vi "Read_CSV_Files_9205x3.vi"() -> ()   [LabVIEW 2018]
uses:
  <vilib>/express/express analysis/Spectral/Block/exnSpectralBlock spectral measurements RMS poly.vi
  <vilib>/express/express analysis/Spectral/Block/exnSpectralBlock spectral measurements RMS DDT.vi
  <vilib>/ErrorRing/Error Ring.xnode
  <vilib>/express/express analysis/Spectral/XNode/ExpressSpectralMeasurementsBlockNode.xnode
panel:
  in  "FFT Mode":bool
  in  "Rechose":bool
  in  "Rescan":bool
  in  "Data Connect":bool
  in  "FFT export":bool
  in  "Filenames":i32(listbox)
  out "error out":errorcluster
  out "Timedomain":dynamicdata(graph)
  out "FFT":dynamicdata(graph)
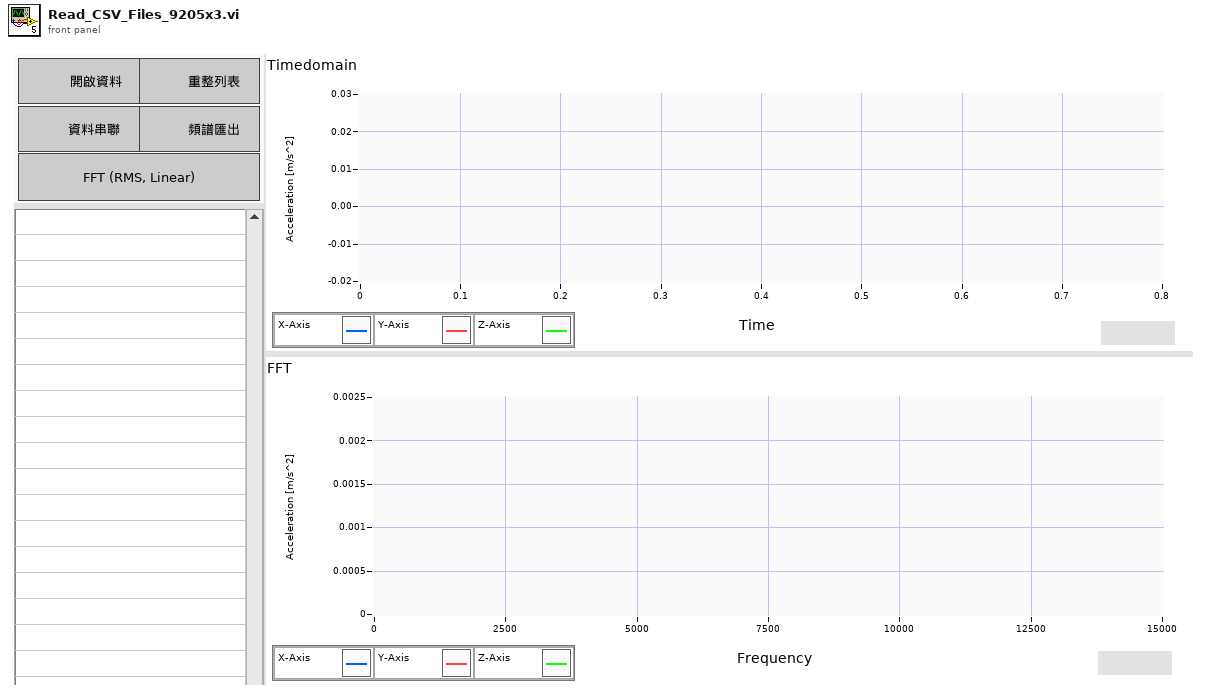
[diagram p1: front panel]
types:
  T1 = cluster{"averaging mode":u16, "weighting mode":u16, "number of averages":u32}
  T2 = cluster{"dB On (F)":bool, "unwrap phase (F)":bool, "convert to degree (F)":bool}
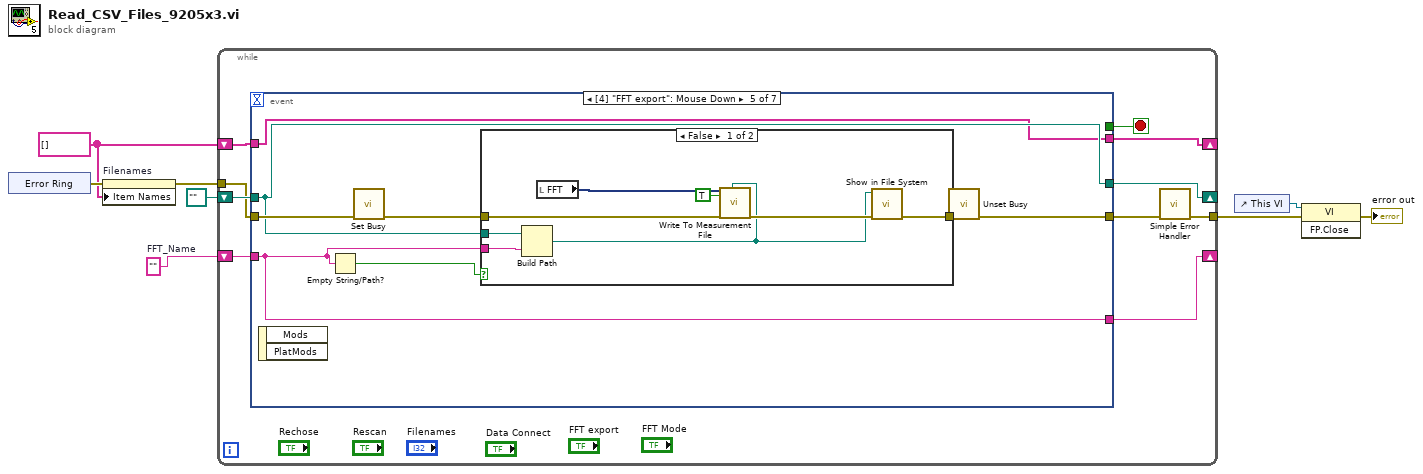
[diagram p0: block diagram]
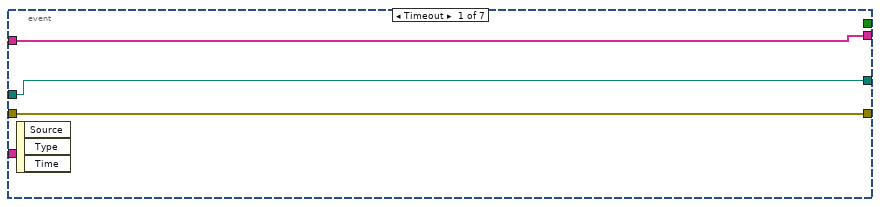
[diagram p2: hidden frame]
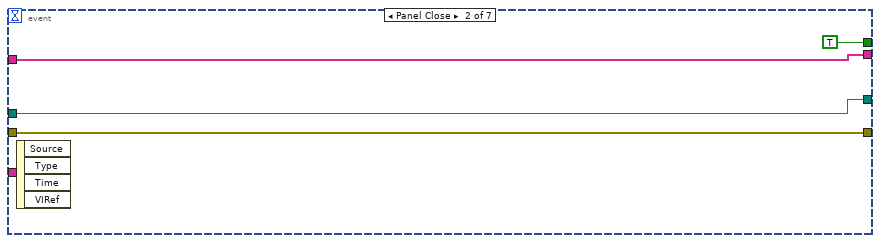
[diagram p3: hidden frame]
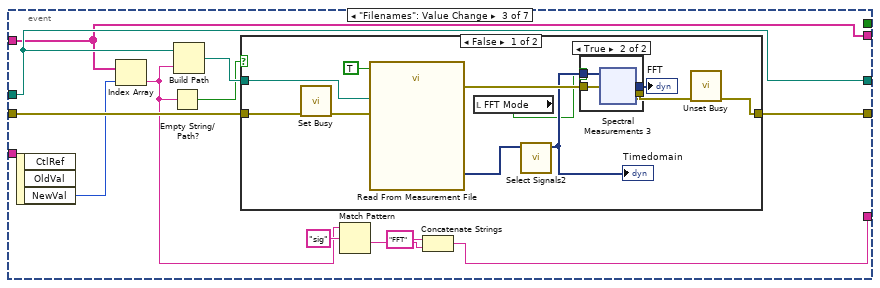
[diagram p4: hidden frame]
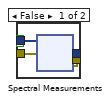
[diagram p5: hidden frame]
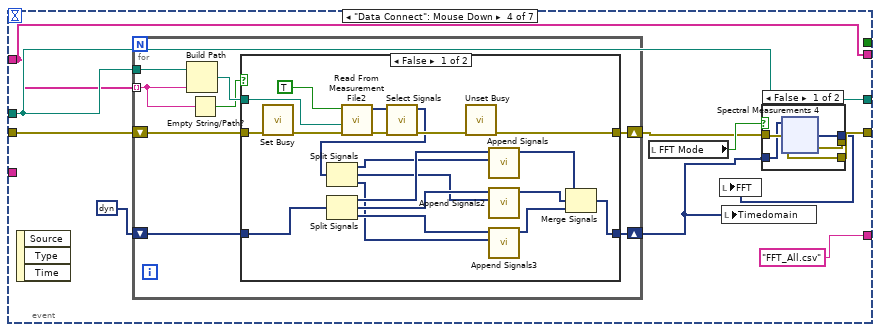
[diagram p7: hidden frame]
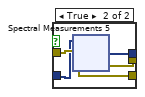
[diagram p8: hidden frame]
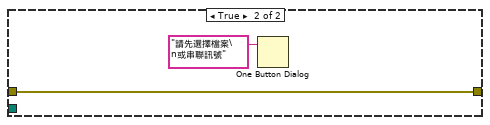
[diagram p10: hidden frame]
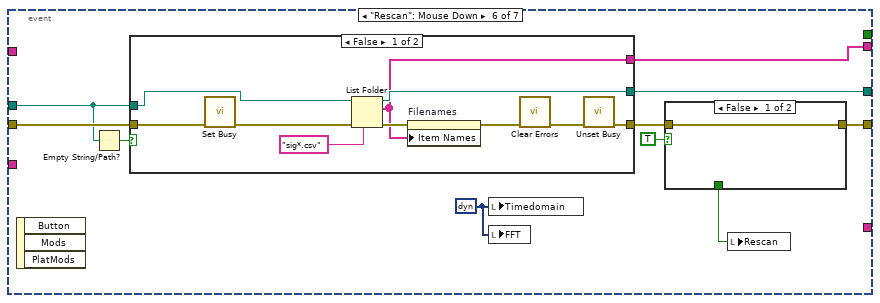
[diagram p11: hidden frame]
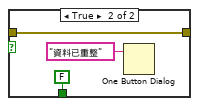
[diagram p12: hidden frame]
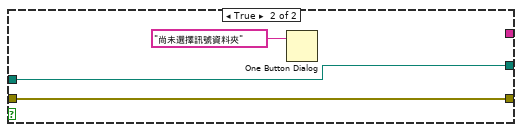
[diagram p13: hidden frame]
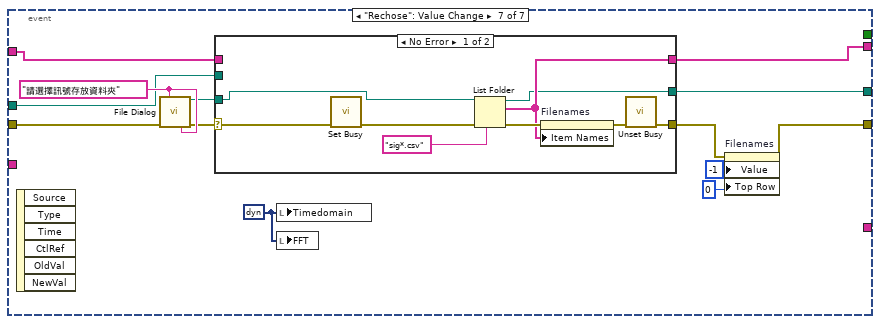
[diagram p14: hidden frame]
diagram:
  w1 = ""  # FFT_Name
  w2 = string[] [] ("filenames")
  n1 = xnode "Error Ring"() -> ("error out"=w4:errorcluster)
  n2 = property on="Filenames" class="LstBox (strict)"(error in=w4, "Item Names"=w2) -> (error out=w3:errorcluster)  [unwired: 1 in, 1 out]
  n3 = while {
    tunnel: [w14] -> w6
    shift-right: [w12] -> _
    shift-left: w2 -> [w16]
    shift-right: [w13] -> _
    shift-left: path "" ("path out") -> [w17]
    tunnel: w3 -> [w11]
    shift-right: [w10] -> _
    shift-left: w1 -> [w9]
    stop <- w18 stop-if-true
    n4 = event shown="[4] \"FFT export\": Mouse Down" {
      selector: _ -> [_ _ _ _ _ _ _]
      dyn-events: _ -> [_ _ _ _ _ _ _]
      timeout: _ -> [_ _ _ _ _ _ _]
      tunnel: [w21 w24 w37 w80 w151 w166 w193] -> w15
      tunnel: [_ TRUE _ _ _ _ _] -> w18
      tunnel: w17 -> [w20 w23 w33 w86 w147 w170 w199]
      tunnel: w16 -> [w19 w22 w32 w85 w146 _ w198]
      tunnel: [w20 w23 w33 w86 w147 w173 w200] -> w13
      tunnel: [w19 w22 w32 w85 w146 w172 w201] -> w12
      tunnel: w11 -> [w21 w24 w34 w87 w153 w171 w196]
      tunnel: [_ _ w27 "FFT_All.csv" w148 _ _] -> w10
      tunnel: w9 -> [_ _ _ _ w148 _ _]
      event Timeout {
        n5 = event-data() -> ()  [unwired: 1 in, 3 out]
      }
      event Panel Close {
        n6 = event-data() -> ()  [unwired: 1 in, 4 out]
      }
      event "Filenames": Value Change {
        n7 = event-data() -> ("NewVal"=w26:i32)  [unwired: 1 in, 2 out]
        n8 = Index Array(array=w32, index=w26) -> (element=w28:string)
        n9 = Empty String/Path?(string/path=w28) -> (empty?=w35:bool)
        n10 = Build Path(base path=w33, name or relative path=w28) -> (appended path=w36:path)
        n11 = case shown="False" w35 {
          tunnel: [w45 w77] -> w37
          tunnel: w36 -> [w48 _]
          tunnel: w34 -> [w44 w77]
          frame False {
            n12 = call <vilib>:"Set Busy.vi"("error in (no error)"=w44) -> ("error out"=w46:errorcluster)  [unwired: 9 in, 1 out]
            n13 = call "Read From Measurement File"("error in (no error)"=w46, "Filename"=w48, "Reset"=TRUE) -> ("error out"=w43:errorcluster, "Signals"=w40:dynamicdata)  [unwired: 3 in, 4 out]
            n14 = local read "FFT Mode"() -> (w38:bool)
            n15 = call "Select Signals2"("Signals"=w40) -> ("Signal Out"=w39:dynamicdata)  [unwired: 9 in, 1 out]
            "Timedomain" <- w39
            n16 = case shown="True" w38 {
              tunnel: w43 -> [w52 w66]
              tunnel: [w51 w65] -> w42
              tunnel: [w50 w64] -> w41
              tunnel: w39 -> [w49 w63]
              frame False {
                n17 = xnode ("Spectral Measurements")("Signals"=w49, "error in (no error)"=w52) -> ("FFT - (RMS)"=w50:dynamicdata, "error out"=w51:errorcluster)  [unwired: 1 out]
              }
              frame True {
                n18 = xnode ("Spectral Measurements 3")("Signals"=w63, "error in (no error)"=w66) -> ("FFT - (RMS)"=w64:dynamicdata, "error out"=w65:errorcluster)  [unwired: 1 out]
              }
            }
            "FFT" <- w41
            n19 = call <vilib>:"Unset Busy.vi"("error in (no error)"=w42) -> ("error out"=w45:errorcluster)  [unwired: 10 in]
          }
          frame True {
          }
        }
        n20 = Match Pattern(string=w28, regular expression="sig") -> (after substring=w30:string)  [unwired: 1 in, 3 out]
        n21 = Concatenate Strings("FFT" ("string"), w30) -> (w27:string)
      }
      event "Data Connect": Mouse Down {
        n22 = event-data() -> ()  [unwired: 1 in, 3 out]
        n23 = for {
          tunnel: w86 -> [w118]
          tunnel: w85 -> [w121] mode=indexing
          shift-right: [w123] -> w81
          shift-left: w87 -> [w119]
          shift-right: [w116] -> w79
          shift-left: dynamicdata [] ("Timedomain 2") -> [w117]
          n24 = Build Path(base path=w118, name or relative path=w121) -> (appended path=w122:path)
          n25 = Empty String/Path?(string/path=w121) -> (empty?=w120:bool)
          n26 = case shown="False" w120 {
            tunnel: [w140 w145] -> w123
            tunnel: w122 -> [w143 _]
            tunnel: w119 -> [w139 w145]
            tunnel: w117 -> [w131 w144]
            tunnel: [w132 w144] -> w116
            frame False {
              n27 = call <vilib>:"Set Busy.vi"("error in (no error)"=w139) -> ("error out"=w141:errorcluster)  [unwired: 9 in, 1 out]
              n28 = Split Signals(w131) -> (w128:dynamicdata, w129:dynamicdata, w130:dynamicdata)  [unwired: 3 in]
              n29 = call "Read From Measurement File2"("error in (no error)"=w141, "Filename"=w143, "Reset"=TRUE) -> ("error out"=w137:errorcluster, "Signals"=w138:dynamicdata)  [unwired: 3 in, 4 out]
              n30 = call "Select Signals"("error in (no error)"=w137, "Signals"=w138) -> ("error out"=w136:errorcluster, "Signal Out"=w127:dynamicdata)  [unwired: 8 in]
              n31 = Split Signals(w127) -> (w126:dynamicdata, w125:dynamicdata, w124:dynamicdata)  [unwired: 3 in]
              n32 = call <vilib>:"Unset Busy.vi"("error in (no error)"=w136) -> ("error out"=w140:errorcluster)  [unwired: 10 in]
              n33 = call "Append Signals"("Input Signal B"=w126, "Input Signal A"=w128) -> ("Appended Signals"=w133:dynamicdata)  [unwired: 8 in, 1 out]
              n34 = call "Append Signals2"("Input Signal B"=w125, "Input Signal A"=w129) -> ("Appended Signals"=w134:dynamicdata)  [unwired: 8 in, 1 out]
              n35 = call "Append Signals3"("Input Signal B"=w124, "Input Signal A"=w130) -> ("Appended Signals"=w135:dynamicdata)  [unwired: 8 in, 1 out]
              n36 = Merge Signals(w133, w134, w135) -> (w132:dynamicdata)
            }
            frame True {
            }
          }
        }
        n37 = local read "FFT Mode"() -> (w82:bool)
        n38 = local write "Timedomain"(w79) -> ()
        n39 = case shown="False" w82 {
          tunnel: [w90 w103] -> _
          tunnel: [w91 w105] -> w78
          tunnel: w81 -> [w89 w104]
          tunnel: [w90 w103] -> w80
          tunnel: w79 -> [w88 w102]
          frame False {
            n40 = xnode ("Spectral Measurements 4")("Signals"=w88, "error in (no error)"=w89) -> ("FFT - (RMS)"=w91:dynamicdata, "error out"=w90:errorcluster)  [unwired: 1 out]
          }
          frame True {
            n41 = xnode ("Spectral Measurements 5")("Signals"=w102, "error in (no error)"=w104) -> ("FFT - (RMS)"=w105:dynamicdata, "error out"=w103:errorcluster)  [unwired: 1 out]
          }
        }
        n42 = local write "FFT"(w78) -> ()
      }
      event "FFT export": Mouse Down {
        n43 = event-data() -> ()  [unwired: 1 in, 2 out]
        n44 = Empty String/Path?(string/path=w148) -> (empty?=w149:bool)
        n45 = call <vilib>:"Set Busy.vi"("error in (no error)"=w153) -> ("error out"=w152:errorcluster)  [unwired: 9 in, 1 out]
        n46 = case shown="False" w149 {
          tunnel: w152 -> [w160 w162]
          tunnel: [w156 w162] -> w150
          tunnel: w147 -> [w155 _]
          tunnel: w148 -> [w159 _]
          frame False {
            n47 = Build Path(base path=w155, name or relative path=w159) -> (appended path=w154:path)
            n48 = local read "FFT"() -> (w161:dynamicdata)
            n49 = call "Write To Measurement File"("Signals"=w161, "Reset"=TRUE, "error in (no error)"=w160, "Filename"=w154) -> ("error out"=w157:errorcluster)  [unwired: 13 in, 2 out]
            n50 = call <vilib>:"Show in File System.vi"("error in (no error)"=w157, "file or directory path"=w154) -> ("error out"=w156:errorcluster)  [unwired: 9 in]
          }
          frame True {
            n51 = One Button Dialog(message="請先選擇檔案\n或串聯訊號") -> ()  [unwired: 1 in, 1 out]
          }
        }
        n52 = call <vilib>:"Unset Busy.vi"("error in (no error)"=w150) -> ("error out"=w151:errorcluster)  [unwired: 10 in]
      }
      event "Rescan": Mouse Down {
        w168 = dynamicdata [] ("Timedomain")
        n53 = event-data() -> ()  [unwired: 1 in, 3 out]
        n54 = Empty String/Path?(string/path=w170) -> (empty?=w169:bool)
        n55 = case shown="False" w169 {
          tunnel: [w185 w188] -> w173
          tunnel: [w184 _] -> w172
          tunnel: [w182 w189] -> w165
          tunnel: w171 -> [w181 w189]
          tunnel: w170 -> [w178 w188]
          frame False {
            n56 = call <vilib>:"Set Busy.vi"("error in (no error)"=w181) -> ("error out"=w183:errorcluster)  [unwired: 9 in, 1 out]
            n57 = List Folder(path=w178, pattern="sig*.csv", error in=w183) -> (path out=w185:path, filenames=w184:string[], error out=w186:errorcluster)  [unwired: 1 in, 1 out]
            n58 = property on="Filenames" class="LstBox (strict)"(error in=w186, "Item Names"=w184) -> (error out=w180:errorcluster)  [unwired: 1 in, 1 out]
            n59 = call <vilib>:"Clear Errors.vi"("error in (no error)"=w180) -> ("error out"=w179:errorcluster)  [unwired: 5 in, 1 out]
            n60 = call <vilib>:"Unset Busy.vi"("error in (no error)"=w179) -> ("error out"=w182:errorcluster)  [unwired: 10 in]
          }
          frame True {
            n61 = One Button Dialog(message="尚未選擇訊號資料夾") -> ()  [unwired: 1 in, 1 out]
          }
        }
        n62 = local write "Timedomain"(w168) -> ()
        n63 = local write "FFT"(w168) -> ()
        n64 = case shown="False" TRUE {
          tunnel: [_ FALSE ("Rescan")] -> w167
          tunnel: [w174 w176] -> w166
          tunnel: w165 -> [w174 w176]
          frame False {
          }
          frame True {
            n65 = One Button Dialog(message="資料已重整") -> ()  [unwired: 1 in, 1 out]
          }
        }
        n66 = local write "Rescan"(w167) -> ()
      }
      event "Rechose": Value Change {
        w191 = dynamicdata [] ("Timedomain")
        w203 = "請選擇訊號存放資料夾" ("prompt")
        n67 = event-data() -> ()  [unwired: 1 in, 6 out]
        n68 = call "File Dialog"("prompt"=w203, "error in"=w196, "pattern label"=w203) -> ("selected path"=w202:path, "error out"=w197:errorcluster)  [unwired: 9 in, 2 out]
        n69 = case shown="No Error" w197 {
          selector: w197 -> [w204 _]
          tunnel: w202 -> [w210 _]
          tunnel: [w209 w213] -> w201
          tunnel: [w208 w214] -> w200
          tunnel: [w205 _] -> w194
          tunnel: w199 -> [_ w214]
          tunnel: w198 -> [_ w213]
          frame No Error {
            n70 = call <vilib>:"Set Busy.vi"("error in (no error)"=w204) -> ("error out"=w206:errorcluster)  [unwired: 9 in, 1 out]
            n71 = List Folder(path=w210, pattern="sig*.csv", error in=w206) -> (path out=w208:path, filenames=w209:string[], error out=w211:errorcluster)  [unwired: 1 in, 1 out]
            n72 = property on="Filenames" class="LstBox (strict)"(error in=w211, "Item Names"=w209) -> (error out=w207:errorcluster)  [unwired: 1 in, 1 out]
            n73 = call <vilib>:"Unset Busy.vi"("error in (no error)"=w207) -> ("error out"=w205:errorcluster)  [unwired: 10 in]
          }
          frame Error {
          }
        }
        n74 = local write "Timedomain"(w191) -> ()
        n75 = local write "FFT"(w191) -> ()
        n76 = property on="Filenames" class="LstBox (strict)"(error in=w194, "Value"=-1 ("Filenames"), "Top Row"=0) -> (error out=w193:errorcluster)  [unwired: 1 in, 1 out]
      }
    }
    n77 = call <vilib>:"Simple Error Handler.vi"("error in (no error)"=w15) -> ("error out"=w14:errorcluster)  [unwired: 4 in, 4 out]
  }
  n78 = control-ref of="This VI"() -> (w7:refnum<vi>)
  n79 = invoke class="VI" method="FP.Close"(reference=w7, error in=w6) -> (error out=→"error out":errorcluster)  [unwired: 1 in, 2 out]
